vi "checkStatus.vi"(8 "error in (no error)":errorcluster, 10 "stop":bool, 11 "Pixelfly in":refnum<class "Pixelfly.lvclass">) -> (0 "error out":errorcluster, 2 "stopped?":bool, 3 "Pixelfly out":refnum<class "Pixelfly.lvclass">)   [LabVIEW 2011, in "Hardware.lvlib" / "Channels.lvlib" / "Pixelfly.lvclass"]
uses:
  Pixelfly.lvclass
  Channels.lvlib
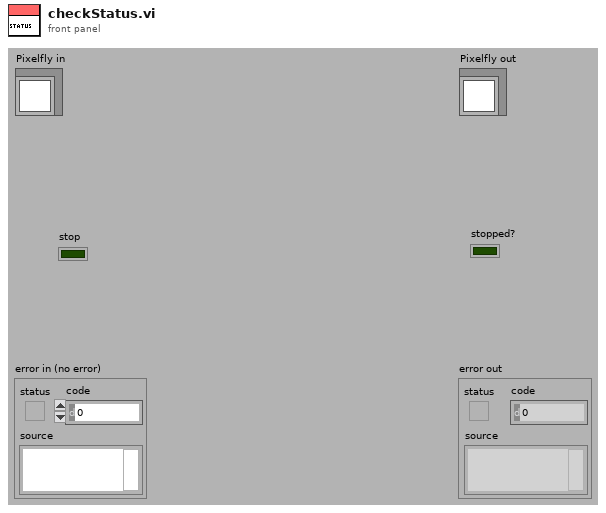
[diagram p1: front panel]
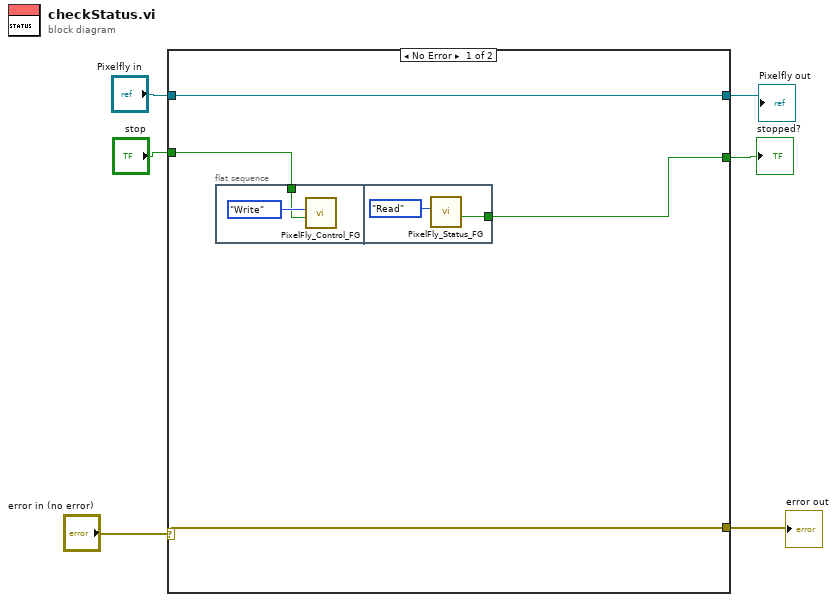
[diagram p0: block diagram]
diagram:
  n1 = case shown="No Error" "error in (no error)" {
    selector: "error in (no error)" -> [w7 w17]
    tunnel: [w7 w17] -> w5
    tunnel: [w10 w16] -> w1
    tunnel: "Pixelfly in" -> [w10 w16]
    tunnel: "stop" -> [w9 w15]
    tunnel: [w8 w15] -> w2
    frame No Error {
      n2 = flat-sequence {
        tunnel: w9 -> [w11]
        tunnel: [w13] -> w8
        frame #0 {
          n3 = call "PixelFly_Control_FG.vi"("stop"=w11, "Action"=enum16{"Write", "Read"}."Write") -> ()  [unwired: 9 in, 1 out]
        }
        frame #1 {
          n4 = call "PixelFly_Status_FG.vi"("Action"=enum16{"Write", "Read"}."Read") -> ("stopped"=w13:bool)  [unwired: 10 in]
        }
      }
    }
    frame Error {
    }
  }
  "error out" <- w5
  "Pixelfly out" <- w1
  "stopped?" <- w2
